vi "Sub_Initialize_LEMP_with_predc.vi"(4 "Handle Fixity":enum16{"Stiffen fixity", "Delete fixty"}(ring), 5 "Effected DOF":i32, 6 "Stiff 2":T1, 7 "Mass 1":T1) -> (0 "Stiff 2":T1, 1 "Natural freq Cantilever pin":dbl[](array[numeric]), 2 "Natural freq Cantilever":dbl[](array[numeric]), 3 "LEMP":T2)   [LabVIEW 2019]
uses:
  <vilib>/Analysis/Matrix/Datatypes/RealMatrix.ctl
  <vilib>/Analysis/7linalg.llb/Real Generalized Eigenvalues and Vectors.vi
  <vilib>/Analysis/Matrix/Numeric/Conversions/Matrix To Array - RM.vi
  <vilib>/Analysis/Matrix/Numeric/Conversions/Array To Matrix - RA2.vi
  <vilib>/Analysis/NI_AALPro.lvlib
  <vilib>/Analysis/Matrix/NI_Matrix.lvlib
panel:
  # "Input"
  # "Output"
  # "This VI acquires the required input cluster for the Sub_online_LEMP_Update.vi, this VI calls on SciPy.linalg.eigh() due to issues with the standard \"General Eigenvalues and Eigenvectors.vi\" outputting inappropriately scaled eigenvectors for the LEMP. Additionally the Bitedness of this installation of LabVIEW does not match with Python so direct python calls were similarly unavailable. The workaround involved a saving the matrices in a text format command line calling the SciPy eigh function saving that output as a text file, then load the output file in to memory (See Sub_Python_cmd_eigh.vi, getEigenCommandPrompt.py , mass.lvm, stiff.lvm,eigenvalues.txt, eigenvectors.txt).\n\n              - Alexander Vereen AFRL Summer scholars 2022"
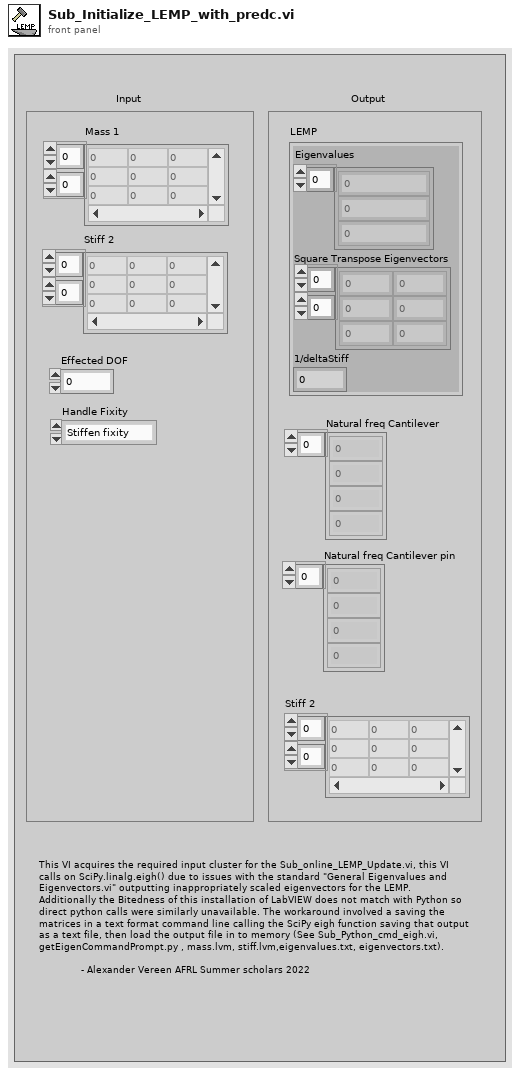
[diagram p1: front panel]
types:
  T1 = typedef "NI_Matrix.lvlib/RealMatrix.ctl" = dbl[][]
  T2 = cluster{"Eigenvalues":dbl[], "Square Transpose Eigenvectors":dbl[][], "1/deltaStiff":dbl}
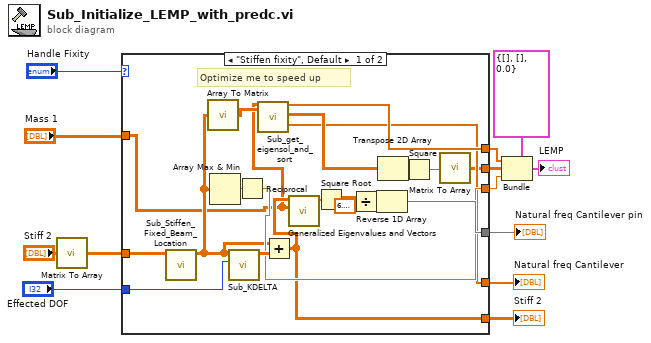
[diagram p0: block diagram]
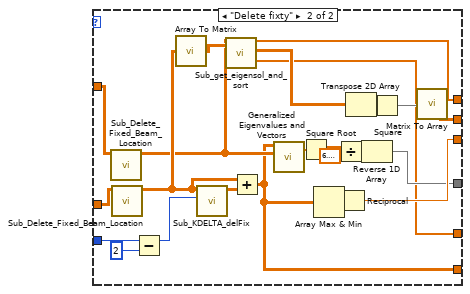
[diagram p2: hidden frame]
diagram:
  n1 = call-poly <vilib>:"Matrix To Array.vi"("Real Matrix"="Stiff 2") -> ("Real 2D Array"=w10:dbl[][])
  n2 = case shown="\"Stiffen fixity\", Default" "Handle Fixity" {
    tunnel: [w28 w44] -> w13
    tunnel: [w27 w43] -> w6
    tunnel: [w17 w42] -> w5
    tunnel: [w22 w45] -> w4
    tunnel: "Mass 1" -> [w14 w38]
    tunnel: "Effected DOF" -> [w21 w46]
    tunnel: w10 -> [w19 w40]
    tunnel: [w18 w41] -> w8
    tunnel: [w15 w36] -> w2
    frame "Stiffen fixity", Default {
      # "Optimize me to speed up"
      n3 = call "Sub_Stiffen_Fixed_Beam_Location.vi"("Pre-BC Matrix"=w19) -> ("Post-BC Matrix"=w16:dbl[][])  [unwired: 10 in]
      n4 = call-poly <vilib>:"Array To Matrix.vi"("Real 2D Array"=w16) -> ("Real Matrix"=w20:T1)
      n5 = Array Max & Min(array=w16) -> (max value=w23:dbl)  [unwired: 3 out]
      n6 = call "Sub_KDELTA.vi"("Pin-Location"=w21, "Pre-Pin Matrix"=w16) -> ("K12"=w25:dbl[][])  [unwired: 8 in]
      n7 = Reciprocal(x=w23) -> (1/x=w22:dbl)
      n8 = call "Sub_get_eigensol_and_sort.vi"("Mass"=w14, "Stiffness"=w20) -> ("Unsorted Eigenvalues"=w27:dbl[], "Unsorted Eigenvector Matrix"=w26:T1, "Natural frequency"=w18:dbl[])  [unwired: 13 in, 2 out]
      n9 = Add(x=w16, y=w25) -> (x+y=w15:dbl[][])
      n10 = call-poly <vilib>:"Generalized Eigenvalues and Vectors.vi"("B"=w14, "A"=w15) -> ("Eigenvalues"=w32:cdb[])  [unwired: 4 in, 2 out]
      n11 = Square Root(x=w32) -> (sqrt(x)=w31:cdb[])
      n12 = Divide(x=w31, y=6.283185307179586) -> (x/y=w29:cdb[])
      n13 = Reverse 1D Array(array=w29) -> (reversed array=w28:cdb[])
      n14 = Transpose 2D Array(2D array=w26) -> (transposed array=w33:T1)
      n15 = Square(x=w33) -> (x^2=w24:T1)
      n16 = call-poly <vilib>:"Matrix To Array.vi"("Real Matrix"=w24) -> ("Real 2D Array"=w17:dbl[][])
    }
    frame "Delete fixty" {
      n17 = call "Sub_Delete_Fixed_Beam_Location.vi"("Pre-BC Matrix"=w38) -> ("Post-BC Matrix"=w37:dbl[][])  [unwired: 10 in]
      n18 = call "Sub_Delete_Fixed_Beam_Location.vi"("Pre-BC Matrix"=w40) -> ("Post-BC Matrix"=w39:dbl[][])  [unwired: 10 in]
      n19 = Subtract(x=w46, y=2) -> (x-y=w35:i32)
      n20 = call-poly <vilib>:"Array To Matrix.vi"("Real 2D Array"=w39) -> ("Real Matrix"=w47:T1)
      n21 = call "Sub_KDELTA_delFix.vi"("Pin-Location"=w35, "Pre-Pin Matrix"=w39) -> ("K12"=w50:dbl[][])  [unwired: 8 in]
      n22 = call "Sub_get_eigensol_and_sort.vi"("Mass"=w37, "Stiffness"=w47) -> ("Unsorted Eigenvalues"=w43:dbl[], "Unsorted Eigenvector Matrix"=w51:T1, "Natural frequency"=w41:dbl[])  [unwired: 13 in, 2 out]
      n23 = Add(x=w39, y=w50) -> (x+y=w36:dbl[][])
      n24 = call-poly <vilib>:"Generalized Eigenvalues and Vectors.vi"("B"=w37, "A"=w36) -> ("Eigenvalues"=w55:cdb[])  [unwired: 4 in, 2 out]
      n25 = Square Root(x=w55) -> (sqrt(x)=w54:cdb[])
      n26 = Array Max & Min(array=w36) -> (max value=w48:dbl)  [unwired: 3 out]
      n27 = Divide(x=w54, y=6.283185307179586) -> (x/y=w52:cdb[])
      n28 = Reciprocal(x=w48) -> (1/x=w45:dbl)
      n29 = Transpose 2D Array(2D array=w51) -> (transposed array=w56:T1)
      n30 = Reverse 1D Array(array=w52) -> (reversed array=w44:cdb[])
      n31 = Square(x=w56) -> (x^2=w49:T1)
      n32 = call-poly <vilib>:"Matrix To Array.vi"("Real Matrix"=w49) -> ("Real 2D Array"=w42:dbl[][])
    }
  }
  "Natural freq Cantilever pin" <- w13
  "Natural freq Cantilever" <- w8
  "Stiff 2" <- w2
  n33 = Bundle(cluster=T2 {"Eigenvalues"=[], "Square Transpose Eigenvectors"=[], "1/deltaStiff"=0.0} ("LEMP"), "Eigenvalues"=w6, "Square Transpose Eigenvectors"=w5, "1/deltaStiff"=w4) -> (→"LEMP":T2)
